vi "Send Load.vi"(5 "Class Relative Paths Path":path, 6 "Loading Method":T1, 7 "Priority":T2=enum."Normal" caption="Message Priority (Normal)", 8 "error in (no error)":errorcluster, 9 "Reference Class Path":path, 10 "Caller Enqueuer":refnum<class "Message Enqueuer.lvclass">, 11 "Message Enqueuer in":refnum<class "Message Enqueuer.lvclass">) -> (0 "error out":errorcluster, 3 "Message Enqueuer out":refnum<class "Message Enqueuer.lvclass">)   [LabVIEW 2023, in "Class Loader.lvlib" / "Load Msg.lvclass"]
doc: "Sends the <b>Load Msg.lvclass</b> message.\n\nThis message will call <b>Load.vi</b> on the <b>Class Loader.lvlib:Class Loader.lvclass</b> actor.\n\n<b>Load.vi Description</b>"
uses:
  Load Msg.lvclass
  Load Msg.lvclass/Load Msg.ctl
  <vilib>/ActorFramework/Message Enqueuer/Message Enqueuer.lvclass
  C:/Program Files/National Instruments/LabVIEW 2023/vi.lib/ActorFramework/Message/Message.lvclass
  C:/Projects/Shared Libraries/Class Loader/Class Loader/Class Loader Messages/Load Msg/Load Msg.lvclass
  <vilib>/ActorFramework/Message Enqueuer/Message Priority.ctl
  Class Loader/Loading Method.ctl
  Class Loader/Class Loader.lvclass
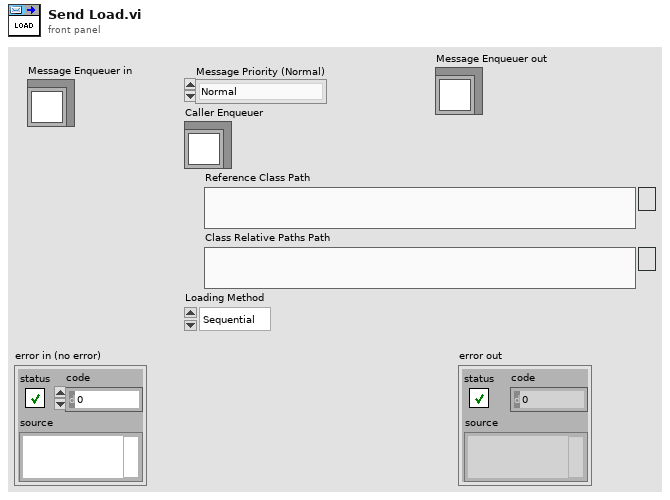
[diagram p1: front panel]
types:
  T1 = typedef "Class Loader.lvlib/Class Loader.lvclass/Loading Method.ctl" = enum16{"Sequential", "Parallel"}
  T2 = typedef "Actor Framework.lvlib/Message Enqueuer.lvclass/Message Priority.ctl" = enum16{"Low", "Normal", "High"}
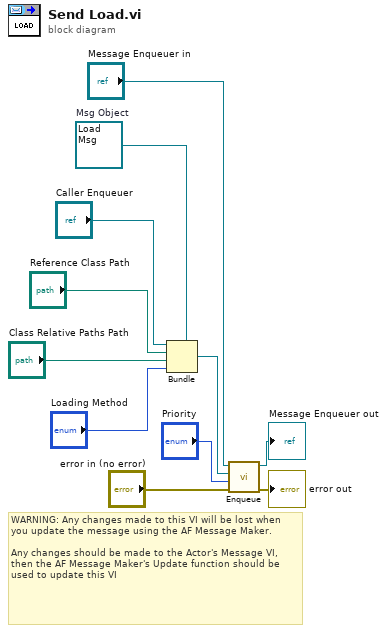
[diagram p0: block diagram]
diagram:
  w7 = refnum<class "Load Msg.lvclass"> refnum  # Msg Object
  # "WARNING: Any changes made to this VI will be lost when you update the message using the AF Message Maker.\n\nAny changes should be made to the Actor's Message VI, then the AF Message Maker's Update function should be used to update this VI"
  n1 = Bundle(cluster=w7, "Caller Enqueuer", "Reference Class Path", "Class Relative Paths Path", "Loading Method") -> (w2:refnum<class "Load Msg.lvclass">)
  n2 = call <vilib>:"Enqueue.vi"("error in (no error)"="error in (no error)", "Message Priority (Normal)"="Priority", "Message"=w2, "Message Enqueuer in"="Message Enqueuer in") -> ("error out"=→"error out":errorcluster, "Message Enqueuer in"=→"Message Enqueuer out":refnum<class "Message Enqueuer.lvclass">)  [unwired: 6 in]
